vi "CRYXY Graph Show.vi"(8 "Frequency Splitter Position":dbl, 11 "pGraph VI":refnum<vi>) -> (2 "XYGarph Ref":refnum<vi>)   [LabVIEW 2013]
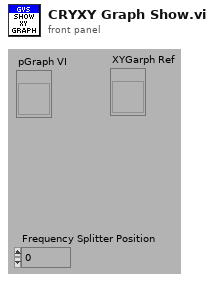
[diagram p1: front panel]
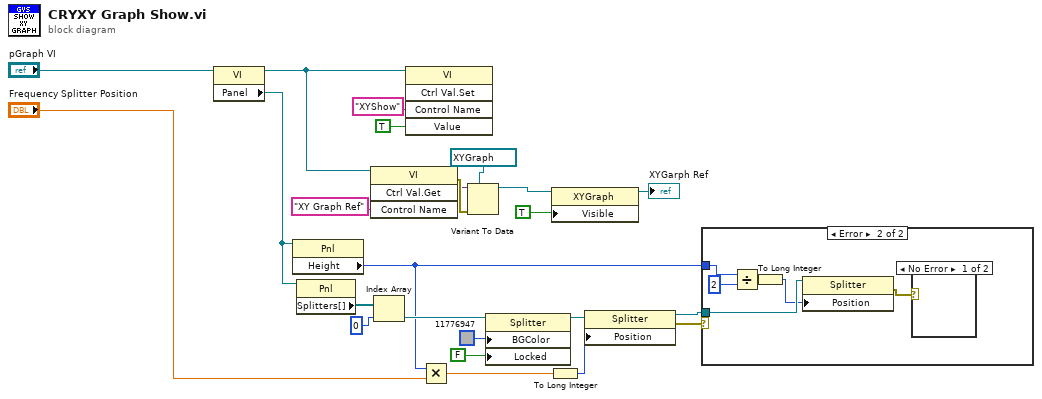
[diagram p0: block diagram]
diagram:
  n1 = property class="VI"(reference="pGraph VI") -> (reference out=w22:refnum<vi>, "Panel"=w21:refnum<vi>)  [unwired: 1 in, 1 out]
  n2 = property class="Pnl"(reference=w21) -> ("Height"=w2:u32)  [unwired: 1 in, 2 out]
  n3 = property class="Pnl"(reference=w21) -> ("Splitters[]"=w12:refnum<vi>[])  [unwired: 1 in, 2 out]
  n4 = invoke class="VI" method="Ctrl Val.Get"(reference=w22, "Control Name"="XY Graph Ref") -> (error out=w18:errorcluster, "Get Control Value Variant"=w17:variant)  [unwired: 2 in, 2 out]
  n5 = Index Array(array=w12, index=0) -> (element=w10:refnum<vi>)
  n6 = invoke class="VI" method="Ctrl Val.Set"(reference=w22, "Control Name"="XYShow", "Value"=TRUE ("Visible")) -> ()  [unwired: 2 in, 5 out]
  n7 = Multiply(x=w2, y="Frequency Splitter Position") -> (x*y=w6:dbl)
  n8 = Variant To Data(error in=w18, type=refnum<vi> refnum ("Legend Ref"), Variant=w17) -> (data=w13:refnum<vi>)  [unwired: 1 out]
  n9 = property on="Property Node" class="Splitter"(reference=w10, "BGColor"=u32 11776947, "Locked"=FALSE ("Splitter Position Locked")) -> (reference out=w7:refnum<vi>)  [unwired: 1 in, 1 out]
  n10 = To Long Integer(number=w6) -> (32bit integer=w5:i32)
  n11 = property class="XYGraph"(reference=w13, "Visible"=TRUE) -> (reference out=→"XYGarph Ref":refnum<vi>)  [unwired: 1 in, 1 out]
  n12 = property on="Property Node" class="Splitter"(reference=w7, "Position"=w5) -> (reference out=w1:refnum<vi>, error out=w3:errorcluster)  [unwired: 1 in]
  n13 = case shown="Error" w3 {
    tunnel: w2 -> [_ w30]
    tunnel: w1 -> [_ w27]
    frame No Error {
    }
    frame Error {
      n14 = Divide(x=w30, y=u32 2) -> (x/y=w28:dbl)
      n15 = To Long Integer(number=w28) -> (32bit integer=w25:i32)
      n16 = property on="Property Node" class="Splitter"(reference=w27, "Position"=w25) -> (error out=w26:errorcluster)  [unwired: 1 in, 1 out]
      n17 = case shown="No Error" w26 {
        frame No Error {
        }
        frame Error {
        }
      }
    }
  }
